vi "Send Initialize card.vi"(7 "Message Priority (Normal)":T2=enum."Normal", 8 "error in (no error)":errorcluster, 9 "Trigger Timeout (10000000)":dbl=1000.0 format="%#_13g", 10 "Control cluster 2":T1={"Number of points"=816000.0, "Input Range"=10000, "Trigger Level"=29, "Trigger source"=TRUE} {"Trigger Level" min=-60 max=60 step=1 scale=-60.0..60.0; "Input Range" items=["+/- 5 V"=10000, "+/- 2 V"=4000, "+/- 1 V"=2000, "+/- 500 mV"=1000, "+/- 200 mV"=400, "+/- 100 mV"=200]; "Number of points" min=160.0 step=160.0}, 11 "Message Enqueuer":refnum<class "Message Enqueuer.lvclass">) -> (0 "error out":errorcluster, 3 "Message Enqueuer out":refnum<class "Message Enqueuer.lvclass">)   [LabVIEW 2015, in "Initialize card Msg.lvclass"]
doc: "This VI sends the message to an actor."
uses:
  Initialize card Msg.lvclass
  <vilib>/ActorFramework/Message Enqueuer/Message Enqueuer.lvclass
  <vilib>/ActorFramework/Message Enqueuer/Message Priority.ctl
  Initialize card Msg.lvclass/Initialize card Msg.ctl
  <vilib>/ActorFramework/Message Enqueuer/Message Enqueuer.lvclass/Message Enqueuer.ctl
  <vilib>/ActorFramework/Message Priority Queue/Priority Enqueue.vi
panel:
  # "Basic Card Controlls"
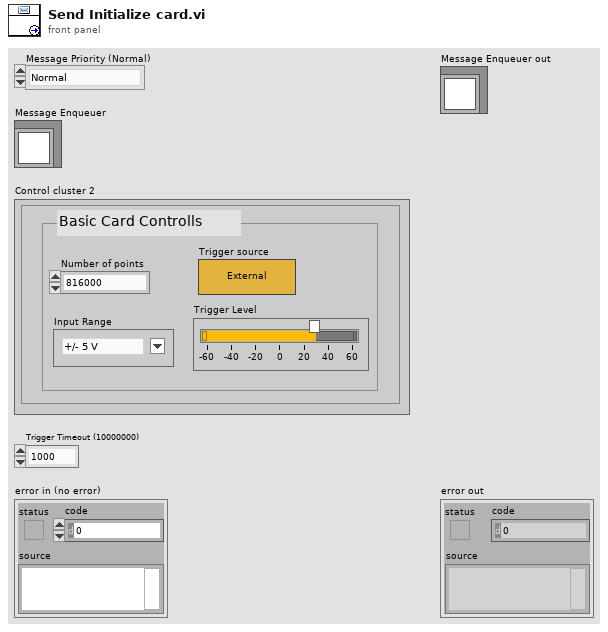
[diagram p1: front panel]
types:
  T1 = cluster{"Number of points":dbl, "Input Range":u32, "Trigger Level":i32, "Trigger source":bool}
  T2 = typedef "Actor Framework.lvlib/Message Enqueuer.lvclass/Message Priority.ctl" = enum16{"Low", "Normal", "High"}
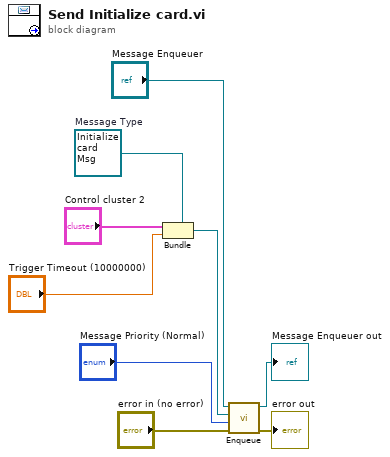
[diagram p0: block diagram]
diagram:
  w6 = refnum<class "Initialize card Msg.lvclass"> refnum  # Message Type
  n1 = Bundle(cluster=w6, "Control cluster 2", "Trigger Timeout (10000000)") -> (w5:refnum<class "Initialize card Msg.lvclass">)
  n2 = call <vilib>:"Enqueue.vi"("error in (no error)"="error in (no error)", "Message Priority (Normal)"="Message Priority (Normal)", "Message"=w5, "Message Enqueuer in"="Message Enqueuer") -> ("error out"=→"error out":errorcluster, "Message Enqueuer out"=→"Message Enqueuer out":refnum<class "Message Enqueuer.lvclass">)  [unwired: 6 in]
